vi "SpectrumAnalyzer.vi"() -> ()   [LabVIEW 2024]
uses:
  <vilib>/express/express analysis/Spectral/Block/exnSpectralBlock spectral measurements RMS poly.vi
  <vilib>/express/express analysis/Spectral/Block/exnSpectralBlock spectral measurements RMS DDT.vi
  <vilib>/express/express analysis/Spectral/Block/exnSpectralBlock spectral measurements power poly.vi
  <vilib>/express/express analysis/Spectral/Block/exnSpectralBlock spectral measurements power DDT.vi
  <vilib>/express/express analysis/Spectral/XNode/ExpressSpectralMeasurementsBlockNode.xnode
panel:
  out "Power Spectrum Graph":dynamicdata(graph)
  out "FFT Waveform Graph":dynamicdata(graph)
  out "Raw Sound":dynamicdata(graph) caption="Data"
  # "Run the program and play a sound that you wish to be analyzed."
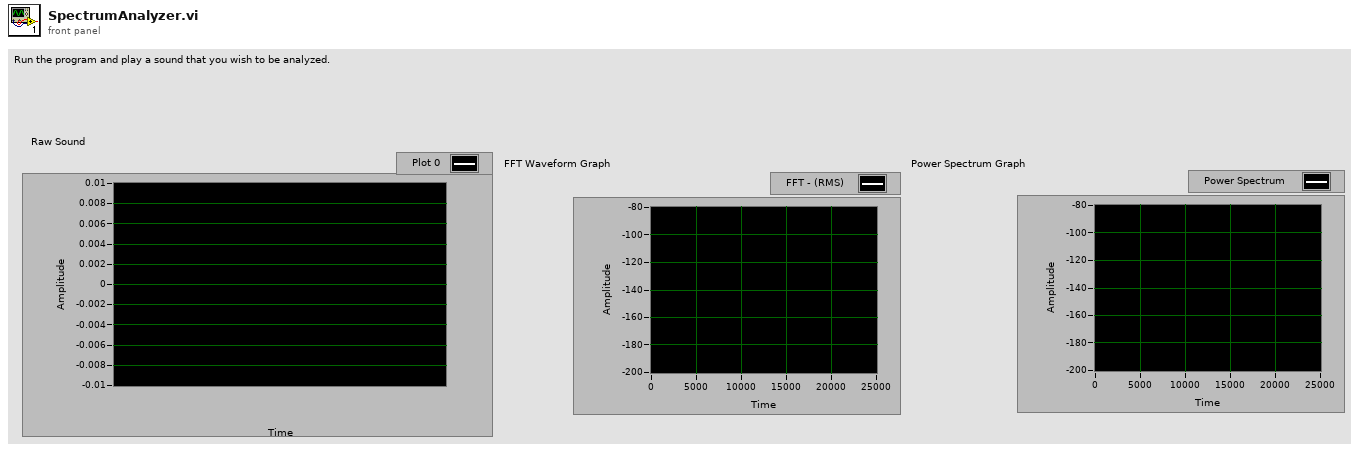
[diagram p1: front panel]
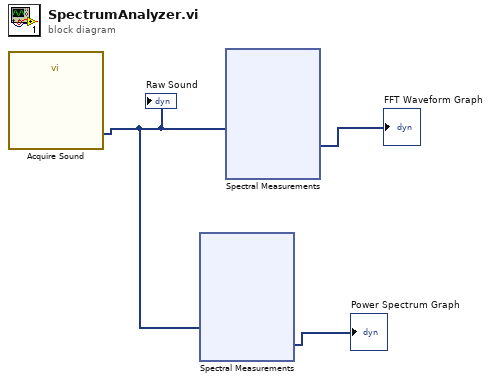
[diagram p0: block diagram]
diagram:
  n1 = call "Acquire Sound"() -> ("Data"=w2:dynamicdata)  [unwired: 18 in, 1 out]
  "Raw Sound" <- w2
  n2 = xnode "Spectral Measurements"("Signals"=w2) -> ("Power Spectrum"=→"Power Spectrum Graph":dynamicdata)  [unwired: 1 in, 1 out]
  n3 = xnode "Spectral Measurements"("Signals"=w2) -> ("FFT - (RMS)"=→"FFT Waveform Graph":dynamicdata)  [unwired: 1 in, 2 out]
